vi "Day02-03.vi"() -> ()   [LabVIEW 2021]
uses:
  b22fa36a-8639-4bed-85e8-8a310910cd56.vi
  929105b9-5548-43d7-acca-99bb8e0b5855.vi
  84a67953-7a4a-431c-bc88-049d6a0513dd.vi
  2f97f8c0-9f97-4a11-a0cb-9674c25bef17.vi
panel:
  out "정렬된 배열":dbl[](array[numeric])
  out "배열":dbl[](array[numeric])
  out "중복 제거된 배열":dbl[](array[numeric]) caption="정렬된 배열"
  out "정렬된 배열":dbl[](array[numeric])
  out "랜덤 난수 값(1~20)":dbl[](array[numeric])
  # "< 문제 >\n  1~20까지의 난수를 10번 발생시키고 정리하며\n중복이 된 부분을 제거하라.\n (배열 + 루프 + 의사결정 구조)"
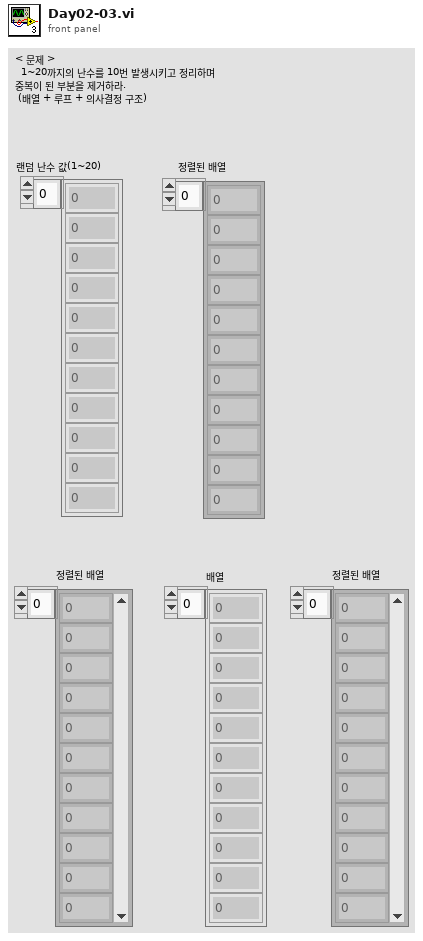
[diagram p1: front panel]
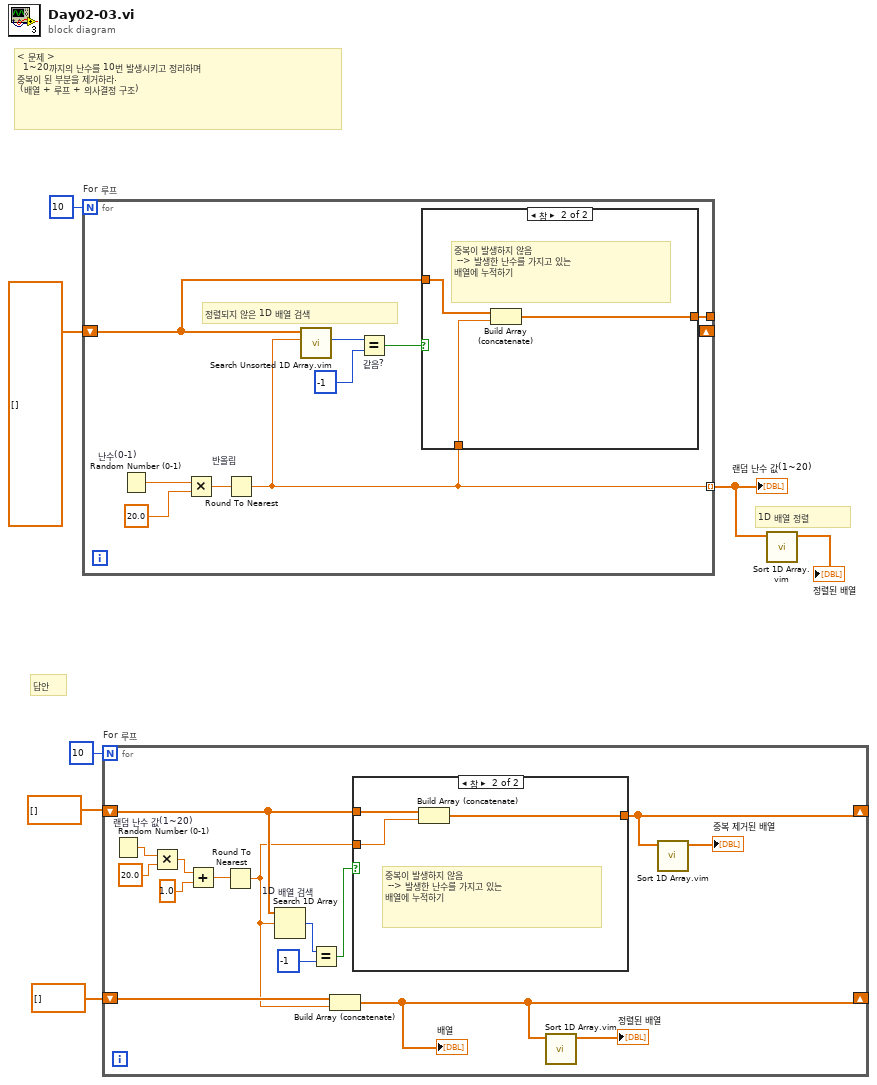
[diagram p0: block diagram]
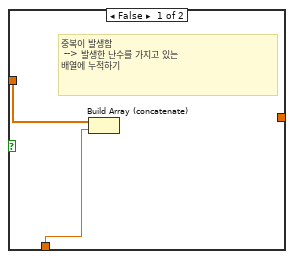
[diagram p3: hidden frame]
diagram:
  # "답안"
  # "1D 배열 정렬"
  # "< 문제 >\n  1~20까지의 난수를 10번 발생시키고 정리하며\n중복이 된 부분을 제거하라.\n (배열 + 루프 + 의사결정 구조)"
  n1 = for "For 루프" {
    N: 10 -> [_]
    tunnel: [w9] -> w6 mode=indexing
    shift-right: _ -> [_]
    shift-left: dbl[] [] -> [w11]
    tunnel: [w8] -> _
    # "정렬되지 않은 1D 배열 검색"
    n2 = Random Number (0-1) "난수(0-1)"() -> (number: 0 to 1=w14:dbl)
    n3 = Multiply(x=w14, y=20.0) -> (x*y=w15:dbl)
    n4 = Round To Nearest "반올림"(number=w15) -> (nearest integer value=w9:dbl)
    n5 = call "Search Unsorted 1D Array.vim"("element"=w9, "unsorted 1D array"=w11) -> ("index of element"=w12:i32)  [unwired: 9 in]
    n6 = Equal? "같음?"(x=w12, y=-1) -> (x = y?=w10:bool)
    n7 = case shown="참" w10 {
      tunnel: w11 -> [w18 w21]
      tunnel: w9 -> [w17 w20]
      tunnel: [_ w19] -> w8
      frame False {
        # "중복이 발생함\n --> 발생한 난수를 가지고 있는\n배열에 누적하기"
        n8 = Build Array (concatenate)(w18, w17) -> ()  [unwired: 1 out]
      }
      frame True {
        # "중복이 발생하지 않음\n --> 발생한 난수를 가지고 있는\n배열에 누적하기"
        n9 = Build Array (concatenate)(w21, w20) -> (w19:dbl[])
      }
    }
  }
  "랜덤 난수 값(1~20)" <- w6
  n10 = for "For 루프" {
    N: 10 -> [_]
    shift-right: [w25] -> _
    shift-left: dbl[] [] -> [w27]
    shift-right: [w23] -> _
    shift-left: dbl[] [] -> [w31]
    n11 = Random Number (0-1) "랜덤 난수 값(1~20)"() -> (number: 0 to 1=w36:dbl)
    n12 = Multiply(x=w36, y=20.0) -> (x*y=w34:dbl)
    n13 = Add(x=w34, y=1.0) -> (x+y=w32:dbl)
    n14 = Round To Nearest(number=w32) -> (nearest integer value=w26:dbl)
    n15 = Search 1D Array "1D 배열 검색"(1D array=w27, element=w26) -> (index of element=w30:i32)  [unwired: 1 in]
    n16 = Equal?(x=w30, y=-1) -> (x = y?=w28:bool)
    n17 = Build Array (concatenate)(w31, w26) -> (w23:dbl[])
    "배열" <- w23
    n18 = case shown="참" w28 {
      tunnel: w27 -> [_ w39]
      tunnel: [_ w38] -> w25
      tunnel: w26 -> [_ w37]
      frame False {
      }
      frame True {
        # "중복이 발생하지 않음\n --> 발생한 난수를 가지고 있는\n배열에 누적하기"
        n19 = Build Array (concatenate)(w39, w37) -> (w38:dbl[])
      }
    }
    n20 = call "Sort 1D Array.vim"("unsorted array"=w23) -> ("sorted array"=→"정렬된 배열":dbl[])  [unwired: 10 in]
    n21 = call "Sort 1D Array.vim"("unsorted array"=w25) -> ("sorted array"=→"중복 제거된 배열":dbl[])  [unwired: 10 in]
  }
  n22 = call "Sort 1D Array.vim"("unsorted array"=w6) -> ("sorted array"=→"정렬된 배열":dbl[])  [unwired: 10 in]
